vi "Get Result.vi"(8 "error in (no error)":errorcluster, 11 "Pulse Driver in":refnum<class "Pulse Driver.lvclass">) -> (0 "error out":errorcluster, 2 "Result":refnum<class "Acquired Result.lvclass">, 3 "Pulse Driver out":refnum<class "Pulse Driver.lvclass">)   [LabVIEW 2015, in "Pulse Driver.lvclass"]
uses:
  Pulse Driver.lvclass
  Measure_core/Results/Acquired Result/Acquired Result.lvclass
  Pulse Driver.lvclass/Pulse Driver.ctl
  Instrument Driver/Instrument Driver.lvclass/Instrument Driver.ctl
  Measure_core/Results/Acquired Result/Acquired Result.lvclass/Acquired Result.ctl
  Read tdms file.vi
  Instrument Driver/Read Channel names.vi
  Measure_core/Results/Acquired Result/Write Finished.vi
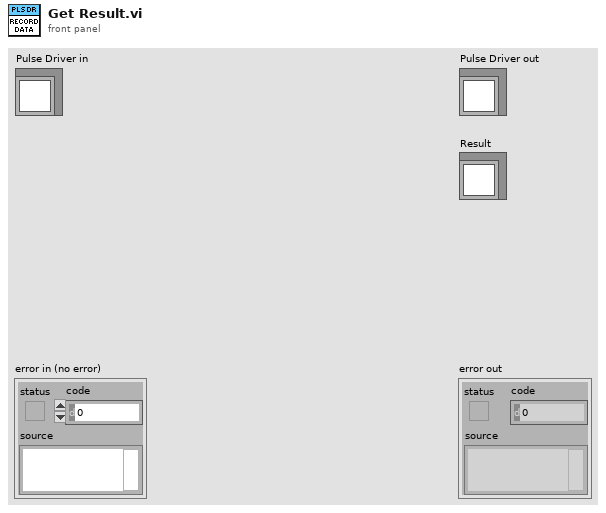
[diagram p1: front panel]
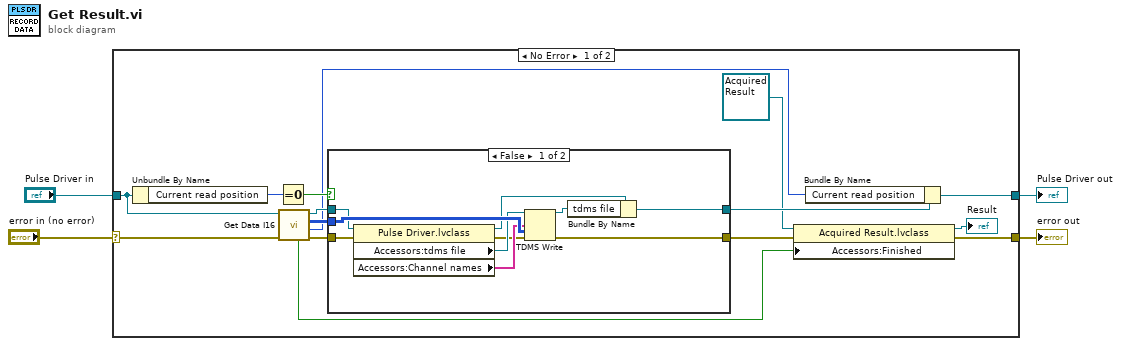
[diagram p0: block diagram]
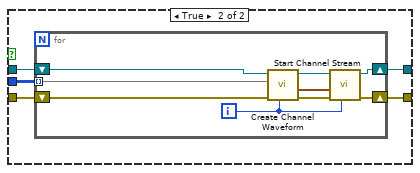
[diagram p2: hidden frame]
diagram:
  n1 = case shown="No Error" "error in (no error)" {
    selector: "error in (no error)" -> [w14 w45]
    tunnel: [w6 w45] -> w3
    tunnel: [w13 w44] -> w1
    tunnel: "Pulse Driver in" -> [w12 w44]
    frame No Error {
      n2 = Unbundle By Name(w12) -> ("Current read position"=w17:i32)
      n3 = Equal To 0?(x=w17) -> (x = 0?=w16:bool)
      n4 = call-dynamic "Get Data I16.vi"("error in (no error)"=w14, "Pulse Driver in"=w12) -> ("error out"=w18:errorcluster, "Current read position"=w10:i32, "Data out"=w15:i16[][], "Pulse Driver out"=w19:refnum<class "Pulse Driver.lvclass">, "Finished"=w7:bool)  [unwired: 5 in]
      n5 = case shown="False" w16 {
        tunnel: w19 -> [w27 w32]
        tunnel: w18 -> [w21 w31]
        tunnel: w15 -> [w29 w34]
        tunnel: [w28 w33] -> w5
        tunnel: [w26 w30] -> w11
        frame False {
          n6 = property class="Pulse Driver.lvclass"(reference=w27, error in=w21) -> (reference out=w24:refnum<class "Pulse Driver.lvclass">, error out=w20:errorcluster, "Accessors:tdms file"=w23:refnum<k34>, "Accessors:Channel names"=w22:string[])
          n7 = TDMS Write(0:w23, 7:w22, 9:w29, 11:w20) -> (4:w25:refnum<k34>, 15:w28:errorcluster)  [unwired: 2 in, 2 out]
          n8 = Bundle By Name(cluster=w24, "tdms file"=w25) -> (w26:refnum<class "Pulse Driver.lvclass">)
        }
        frame True {
          n9 = for {
            tunnel: w34 -> [w40] mode=indexing
            shift-right: [w37] -> w33
            shift-left: w31 -> [w38]
            shift-right: [w41] -> w30
            shift-left: w32 -> [w42]
            i -> [w39]
            n10 = call-dynamic "Create Channel Waveform.vi"("Channel index"=w39, "error in (no error)"=w38, "Data"=w40, "Pulse Driver in"=w42) -> ("error out"=w36:errorcluster, "Waveform out"=w35:waveform(i16), "Pulse Driver out"=w43:refnum<class "Pulse Driver.lvclass">)  [unwired: 5 in]
            n11 = call-dynamic "Start Channel Stream.vi"("Channel index"=w39, "error in (no error)"=w36, "Waveform"=w35, "Pulse Driver in"=w43) -> ("error out"=w37:errorcluster, "Pulse Driver out"=w41:refnum<class "Pulse Driver.lvclass">)  [unwired: 6 in]
          }
        }
      }
      n12 = property class="Acquired Result.lvclass"(reference=refnum<class "Acquired Result.lvclass"> refnum ("Result"), error in=w5, "Accessors:Finished"=w7) -> (reference out=→"Result":refnum<class "Acquired Result.lvclass">, error out=w6:errorcluster)
      n13 = Bundle By Name(cluster=w11, "Current read position"=w10) -> (w13:refnum<class "Pulse Driver.lvclass">)
    }
    frame Error {
    }
  }
  "error out" <- w3
  "Pulse Driver out" <- w1
